vi "calc_focus_test.vi"() -> ()   [LabVIEW 2023]
uses:
  Vision.lvlib
panel:
  in  "File Path":path=path "C:/Users/Caleb/Desktop/obama.jpg"
  out "focus":sgl
  out "error out":errorcluster
  out "Image":T1(plugin-control)
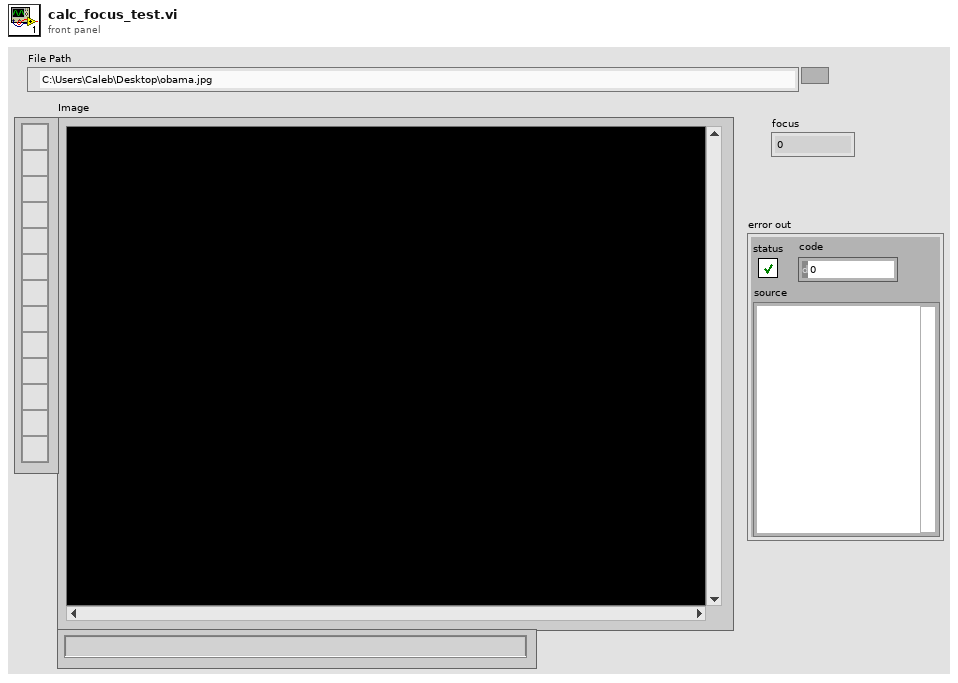
[diagram p1: front panel]
types:
  T1 = typedef "IMAQ Image.ctl" = refnum<image>
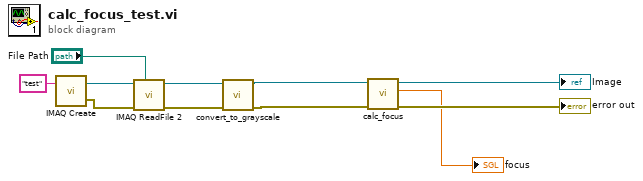
[diagram p0: block diagram]
diagram:
  n1 = call "IMAQ Create"("Image Name"="test") -> ("New Image"=w11:T1, "error out"=w9:errorcluster)  [unwired: 4 in]
  n2 = call "IMAQ ReadFile 2"("File Path"="File Path", "error in (no error)"=w9, "Image"=w11) -> ("error out"=w4:errorcluster, "Image Out"=w5:T1)  [unwired: 4 in, 3 out]
  n3 = call "convert_to_grayscale.vi"("error in (no error)"=w4, "Image in"=w5) -> ("error out"=w3:errorcluster, "Image out"=w2:T1)  [unwired: 8 in]
  n4 = call "calc_focus.vi"("error in"=w3, "Image"=w2) -> ("error out"=→"error out":errorcluster, "focus"=→"focus":sgl, "Image out"=→"Image":T1)  [unwired: 7 in]
